vi "Cell TDMS fit and purge MAIN mask v2a BigImage HEATHER 8Bit.vi"() -> ()   [LabVIEW 2020]
uses:
  <vilib>/Utility/file.llb/Read Delimited Spreadsheet (I64).vi
  <vilib>/Utility/file.llb/Write Delimited Spreadsheet (DBL).vi
  <vilib>/Analysis/1siggen.llb/Ramp Pattern by Delta.vi
  <vilib>/Analysis/NI_AALBase.lvlib
  <vilib>/Analysis/NI_AALPro.lvlib
panel:
  in  "Save as binary?":bool
  in  "Min size":u16=400
  out "low threshold":dbl
  in  "threshold 2":dbl(knob)=0.2050666550953167 scale=0.0..1.0
  in  "Save mask?":bool
  in  "WRITE: tiff mask":path=path "F:/Andrey/Heather puncta/Heather mask.tif"
  in  "WRITE: file path to save low/high threshold":path=path "F:/Andrey/Heather puncta/Heather low high threshold.lvm"
  in  "WRITE: file path to save corrected results":path=path "F:/Andrey/Heather puncta/Heather corrected results.lvm"
  in  "Exclude puncta?":bool
  in  "Save centroid results?":bool
  in  "WRITE: file path to save centroid results":path=path "F:/Andrey/Heather puncta/Heather centroid result.lvm"
  out "Fit result picture":picture
  in  "Save PNG?":bool
  in  "WRITE: Fit result save path":path=path "F:/Andrey/Heather puncta/Heather line fit to ave.png"
  out "Fit to data":cluster{"Ramp Pattern":dbl[], dbl[]}[](graph)
  in  "Save corrected?":bool
  in  "WRITE: corrected data file":path=path "F:/Andrey/Heather puncta/Heather cell corrected.tif"
  out "size(s)":i32[](array[numeric])
  in  "Save results?":bool
  in  "WRITE: file path to save results":path=path "F:/Andrey/Heather puncta/Heather results.lvm"
  in  "Use mask?":bool
  in  "READ: Folder/file path for individual cell(s) signal":path=path "E:/WORK/Ehrhardt Lab/Heather Meyer/Txt files for Andrey/phm5S-SUF4 5S variant 4/phm5S_4_cell1"
  out "filename":string
  out "sum":u32
  out "Histogram Graph":T1(graph)
  out "Mask":u8[][](graph)
  out "high threshold":u16
  out "Binarized":u8[][](graph)
  out "new picture (in 8 bit for visualization only)":picture
  in  "Data format?":i8(knob)=1 scale=0.0..2.0
  in  "threshold":dbl(knob)=0.2050666550953167 scale=0.0..1.0
  # "Use mask ON = keep only centroid\nExclude puncta ON = puncta EXCLUDED for the purpose of \ncalculating the curve for image normalization\nCorrected image is cropped by mask INCLUDING puncta,\nregardless of this selector"
  # "txt"
  # "Select file (1 cell only) or folder (for batch processing):"
  # "Version 2.5\nAVM"
  # "120 should be good"
  # "binary"
  # "tiff"
  # "Raw data"
  # "(x100% of max value)"
  # "200-600"
  # "Single Z-section to\nshow for visualization."
  # "Values of intensity for every pixel"
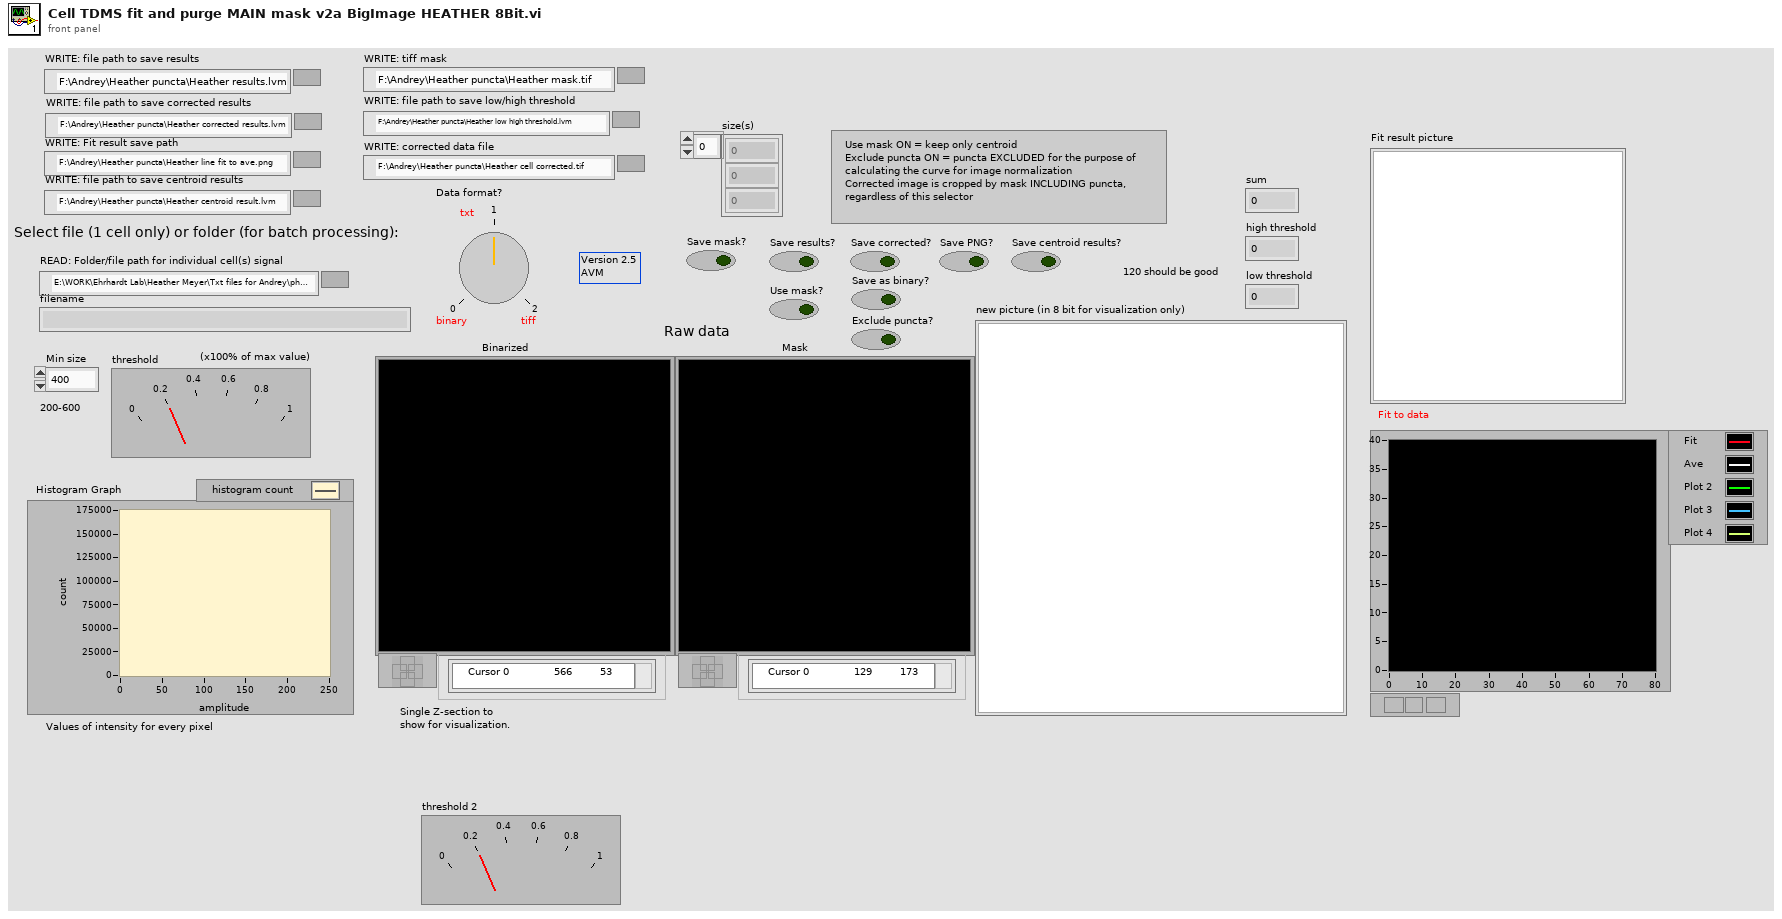
[diagram p1: front panel]
types:
  T1 = cluster{"X Values":dbl[], "Histogram: h(x)":i32[]}
  T2 = cluster{"Width":u16, "Style":enum32{"Solid", "Dash", "Dot", "DashDot", "DashDotDot"}}
  T3 = typedef "imagedata.ctl" = cluster{"image type":i32, "image depth":i32, "image":u8[], "mask":u8[], "colors":u32[], "Rectangle":cluster{"left":i16, "top":i16, "right":i16, "bottom":i16}}
  T4 = typedef "Image Type" = u32
  T5 = typedef "IMAQ Image.ctl" = refnum<image>
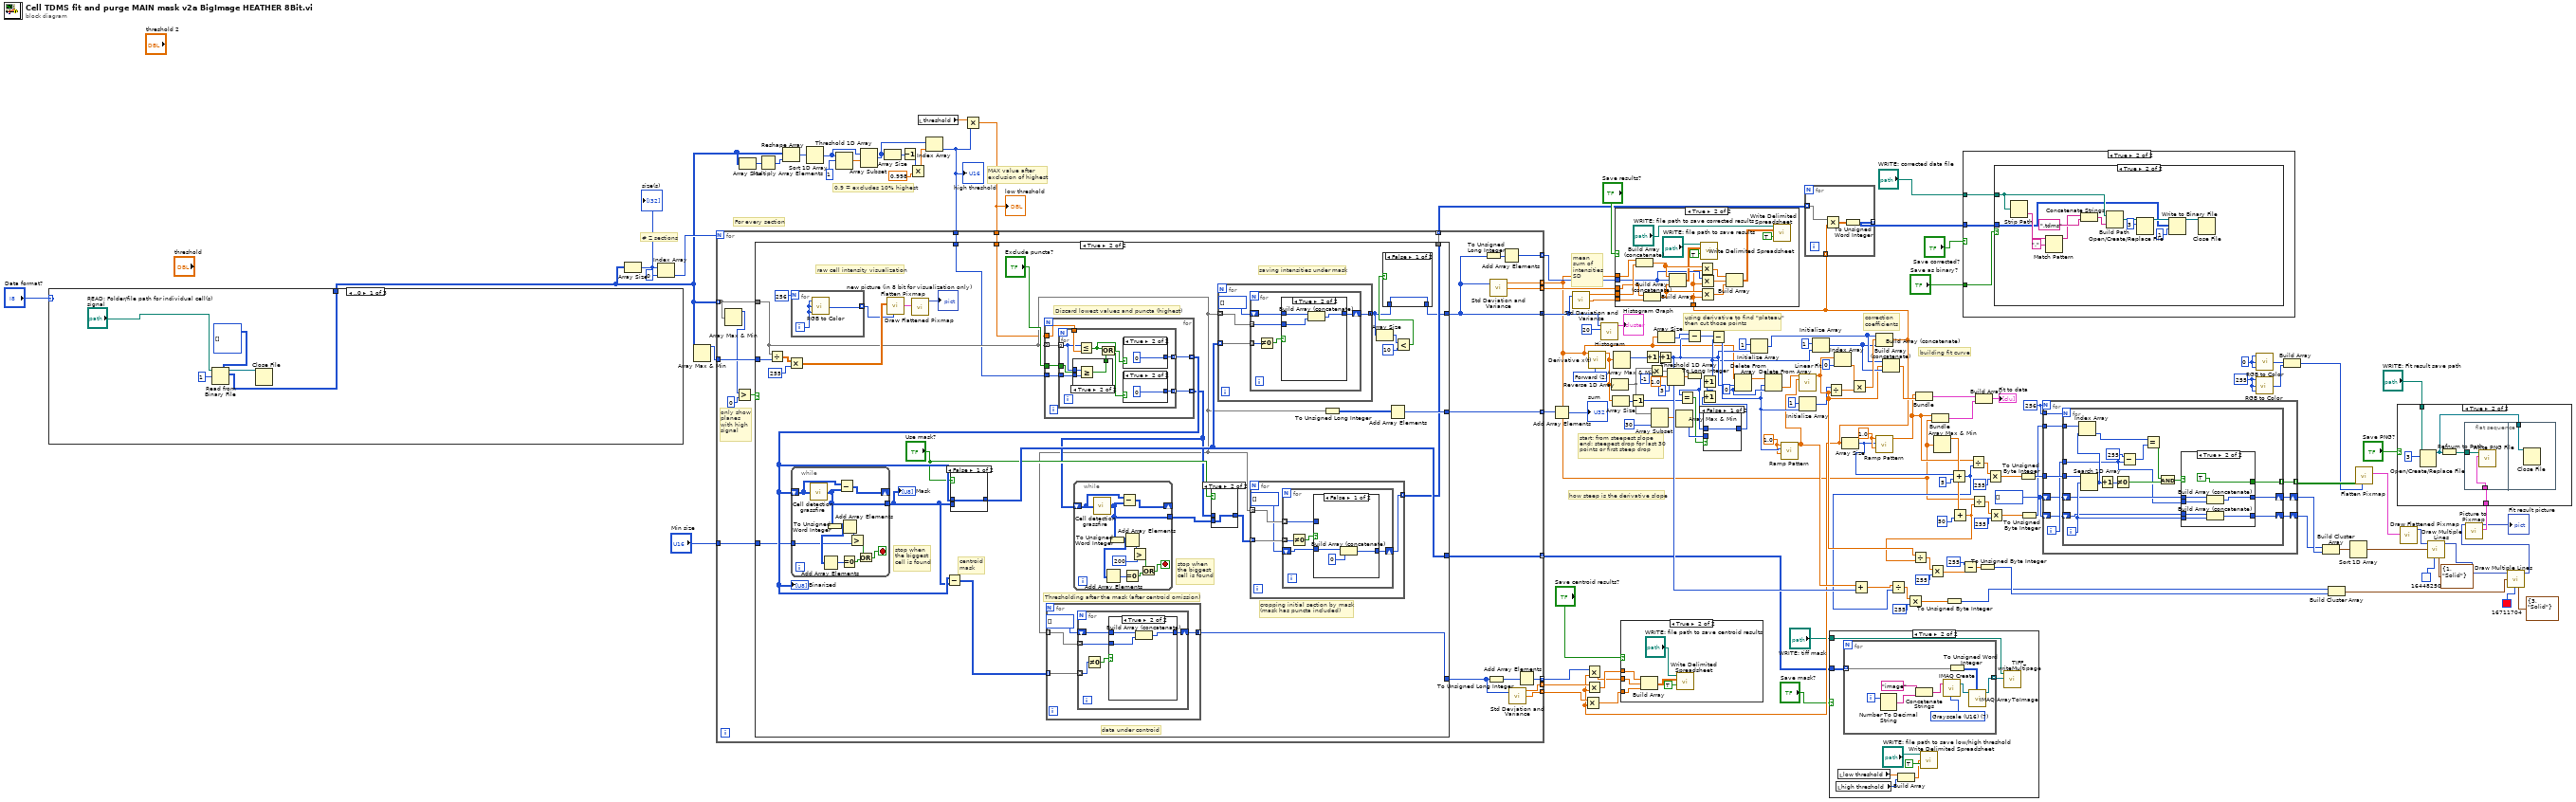
[diagram p0: block diagram]
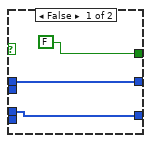
[diagram p5: hidden frame]
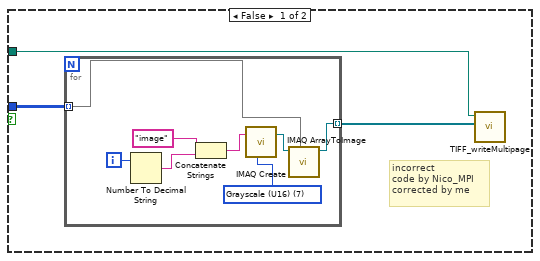
[diagram p8: hidden frame]
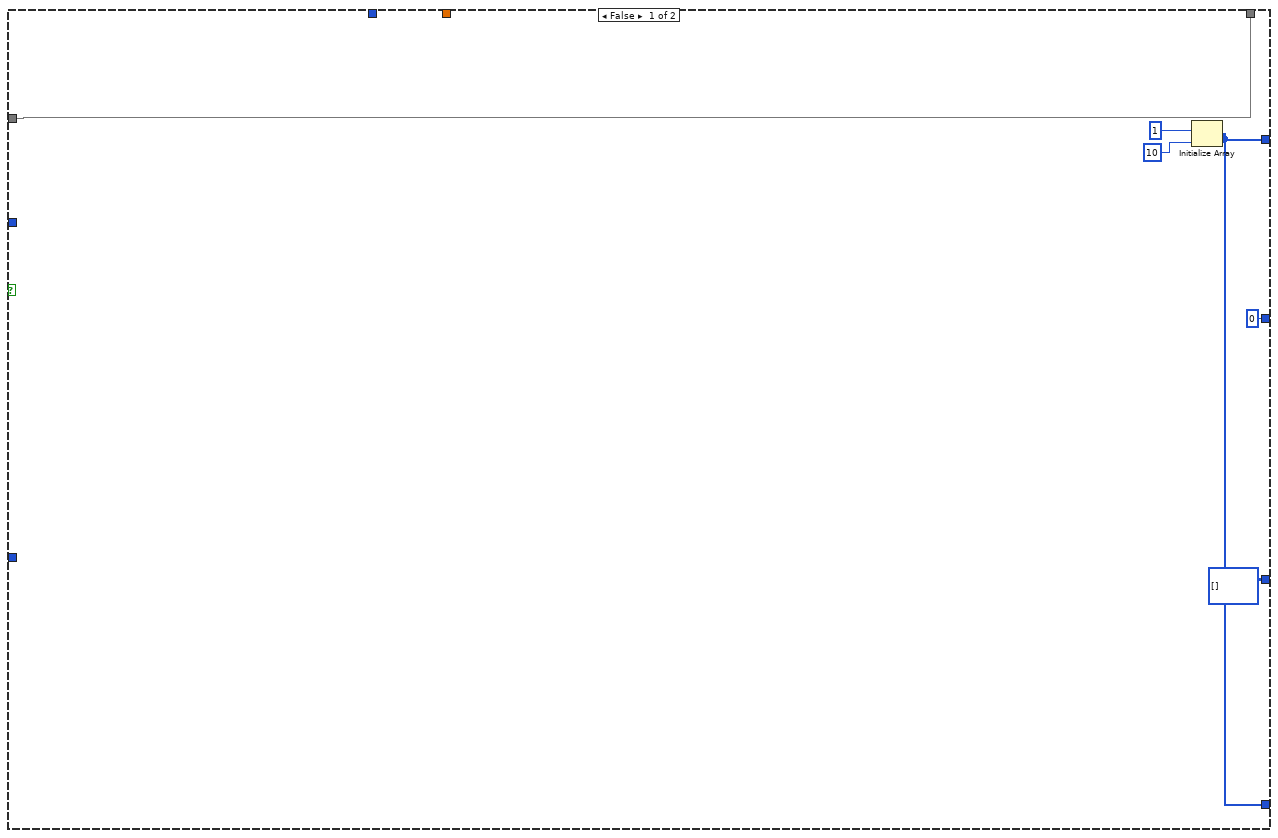
[diagram p10: hidden frame]
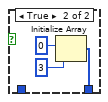
[diagram p11: hidden frame]
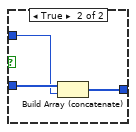
[diagram p12: hidden frame]
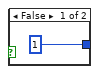
[diagram p17: hidden frame]
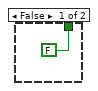
[diagram p18: hidden frame]
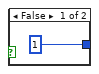
[diagram p19: hidden frame]
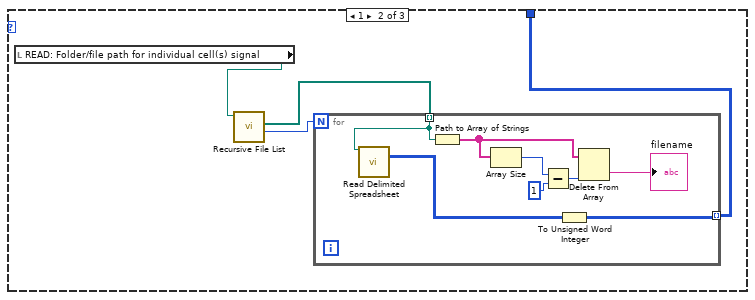
[diagram p20: hidden frame]
diagram:
  w88 = i32[] []
  w66 = u8 255 ("index (row)")
  w78 = u8 0 ("index (row)")
  w95 = 256
  w114 = 1.0 ("delta")
  w117 = 1.0 ("delta")
  w121 = 0 ("index")
  w132 = u16 2 items=["2nd Order Central", "4th Order Central", "Forward", "Backward"] ("method")
  # "building fit curve"
  # "how steep is the derivative slope"
  # "MAX value after\nexclusion of highest"
  # "0.9 = excludes 10% highest"
  # "start: from steepest slope\nend: steepest drop for last 30\npoints or first steep drop"
  # "correction\ncoefficients"
  # "using derivative to find \"plateau\"\nthen cut those points"
  # "For every section"
  # "mean\nsum of\nintensities\nSD"
  # "# Z sections"
  n1 = case shown="..0" "Data format?" {
    tunnel: [w146 w151 w163] -> w9
    frame ..0 {
      n2 = Read from Binary File(5:u8[][][] [] ("subarray"), 9:1, 11:"READ: Folder/file path for individual cell(s) signal") -> (2:w146:u8[][][], 3:w149:refnum<file>)  [unwired: 3 in, 2 out]
      n3 = Close File(refnum=w149) -> ()  [unwired: 1 in, 2 out]
    }
    frame 1 {
      n4 = local read "READ: Folder/file path for individual cell(s) signal"() -> (w150:path)
      n5 = call <vilib>:"Recursive File List.vi"("Folder Path"=w150) -> ("Number of Files"=w153:i32, "All Files in Dir"=w152:path[])  [unwired: 6 in, 3 out]
      n6 = for {
        N: w153 -> [_]
        tunnel: w152 -> [w160] mode=indexing
        tunnel: [w155] -> w151 mode=indexing
        n7 = call-poly <vilib>:"Read Delimited Spreadsheet.vi"("file path (dialog if empty)"=w160) -> ("all rows"=w154:i64[][])  [unwired: 9 in, 5 out]
        n8 = Path to Array of Strings(0:w160) -> (2:w161:string[])  [unwired: 1 out]
        n9 = Array Size(array=w161) -> (size(s)=w156:i32)
        n10 = Subtract(x=w156, y=1 ("index (row)")) -> (x-y=w157:i32)
        n11 = To Unsigned Word Integer(number=w154) -> (unsigned 16bit integer=w155:u16[][])
        n12 = Delete From Array(array=w161, index=w157) -> (deleted portion=→"filename":string)  [unwired: 1 in, 1 out]
      }
    }
    frame 2.. {
      n13 = local read "READ: Folder/file path for individual cell(s) signal"() -> (w164:path)
      n14 = call "Load 3D tiff stack.vi"("Image File"=w164) -> ("24-bit pixmap"=w162:u32[][][])
      n15 = To Unsigned Word Integer(number=w162) -> (unsigned 16bit integer=w163:u16[][][])
    }
  }
  n16 = Array Size(array=w9) -> (size(s)=w143:i32[])
  "size(s)" <- w143
  n17 = Index Array(array=w143, index=0) -> (element=w138:i32)
  n18 = Array Max & Min(array=w9) -> (max value=w139:u16)  [unwired: 3 out]
  n19 = Array Size(array=w9) -> (size(s)=w12:i32[])
  n20 = Multiply Array Elements(1:w12) -> (0:w11:i32)
  n21 = Reshape Array(w9, w11) -> (w16:u16[])
  n22 = Sort 1D Array(array=w16) -> (sorted array=w15:u16[])
  n23 = Threshold 1D Array(2:i16 1 ("y"), 3:w15) -> (0:w17:dbl)  [unwired: 1 in]
  n24 = Array Subset(array=w15, index=w17) -> (w14:u16[])  [unwired: 1 in]
  n25 = Array Size(array=w14) -> (size(s)=w19:i32)
  n26 = Decrement(x=w19) -> (x-1=w18:i32)
  n27 = Multiply(x=w18, y=0.998) -> (x*y=w20:dbl)
  n28 = local read "threshold"() -> (w10:dbl)
  n29 = Index Array(array=w14, index=w20) -> (element=w7:u16)
  "high threshold" <- w7
  n30 = Multiply(x=w10, y=w7) -> (x*y=w8:dbl)
  "low threshold" <- w8
  n31 = for {
    N: w138 -> [_]
    tunnel: [w166] -> w39 mode=concatenating
    tunnel: w139 -> [w185]
    tunnel: w9 -> [w184] mode=indexing
    tunnel: [w180] -> w6 mode=indexing
    tunnel: [w179] -> w136 mode=indexing
    tunnel: [w177] -> w135 mode=indexing
    tunnel: [w176] -> w134 mode=indexing
    tunnel: [w174] -> w38 mode=indexing
    tunnel: [w172] -> w48 mode=indexing
    tunnel: [w171] -> w49 mode=indexing
    tunnel: [w170] -> w35 mode=indexing
    tunnel: [w169] -> w33 mode=indexing
    tunnel: w8 -> [w168]
    tunnel: w7 -> [w167]
    tunnel: "Min size" -> [w165]
    # "only show\nplanes\nwith high\nsignal"
    n32 = Array Max & Min(array=w184) -> (max value=w181:u16)  [unwired: 3 out]
    n33 = Greater?(x=w181, y=i16 0) -> (0:w183:bool)
    n34 = case shown="True" w183 {
      tunnel: [w189 w193] -> w166
      tunnel: w185 -> [_ w214]
      tunnel: w184 -> [w187 w201]
      tunnel: [u16 0 ("index (row)") w213] -> w176
      tunnel: [w189 w210] -> w173
      tunnel: [w187 w203] -> w170
      tunnel: [u8[][] [] ("Cell") w207] -> w169
      tunnel: w168 -> [_ w200]
      tunnel: w167 -> [_ w199]
      tunnel: w165 -> [_ w192]
      frame False {
        n35 = Initialize Array(u16 1 ("index (row)"), u8 10 ("index (row)")) -> (w189:u16[])
      }
      frame True {
        # "cropping initial section by mask\n(mask has puncta included)"
        # "stop when\nthe biggest\ncell is found"
        # "data under controid"
        # "centroid\nmask"
        # "Thresholding after the mask (after centroid omission)"
        # "Discard lowest values and puncta (highest)"
        # "stop when\nthe biggest\ncell is found"
        # "raw cell intensity visualization"
        # "saving intensities under mask"
        n36 = Divide(x=w201, y=w214) -> (x/y=w221:dbl[][])
        n37 = Multiply(x=w221, y=i16 255) -> (x*y=w220:dbl[][])
        n38 = for {
          N: 256 ("samples") -> [_]
          tunnel: [w314] -> w217 mode=indexing
          i -> [w315]
          n39 = call <vilib>:"RGB to Color.vi"("B"=w315, "G"=w315, "R"=w315) -> ("Color"=w314:u32)
        }
        n40 = call <vilib>:"Flatten Pixmap.vi"("colors"=w217, "8-bit pixmap"=w220) -> ("image data"=w216:T3)  [unwired: 9 in]
        n41 = call <vilib>:"Draw Flattened Pixmap.vi"("image data"=w216) -> ("new picture"=→"new picture (in 8 bit for visualization only)":picture)  [unwired: 8 in]
        n42 = for {
          tunnel: [w296] -> w212 mode=indexing
          tunnel: w201 -> [w295] mode=indexing
          tunnel: w200 -> [w294]
          tunnel: w199 -> [w293]
          tunnel: "Exclude puncta?" -> [w292]
          tunnel: [w291] -> w205 mode=indexing
          n43 = for {
            tunnel: w295 -> [w300] mode=indexing
            tunnel: [w305] -> w296 mode=indexing
            tunnel: w294 -> [w304]
            tunnel: w293 -> [w301]
            tunnel: w292 -> [w299]
            tunnel: [w297] -> w291 mode=indexing
            n44 = case shown="True" w299 {
              tunnel: [FALSE w311] -> w303
              tunnel: w301 -> [_ w310]
              tunnel: w300 -> [_ w309]
              frame False {
              }
              frame True {
                n45 = Greater Or Equal?(x=w309, y=w310) -> (x >= y?=w311:bool)
              }
            }
            n46 = Less Or Equal?(x=w300, y=w304) -> (x <= y?=w298:bool)
            n47 = Or(x=w298, y=w303) -> (x .or. y?=w302:bool)
            n48 = case shown="True" w302 {
              tunnel: [u8 1 ("index (row)") u8 0 ("index (row)")] -> w305
              frame False {
              }
              frame True {
              }
            }
            n49 = case shown="True" w298 {
              tunnel: [u8 1 ("index (row)") u8 0 ("index (row)")] -> w297
              frame False {
              }
              frame True {
              }
            }
          }
        }
        "Binarized" <- w212
        n50 = while {
          shift-right: [w276] -> _
          shift-left: w212 -> [w277]
          tunnel: [w274] -> w209
          tunnel: w192 -> [w268]
          stop <- w272 stop-if-true
          n51 = call "Cell detection grassfire.vi"("Intensities"=w277) -> ("Cell"=w274:u8[][])
          n52 = To Unsigned Word Integer(number=w274) -> (unsigned 16bit integer=w269:u16[][])
          n53 = Add Array Elements(numeric array=w269) -> (sum=w270:u16)
          n54 = Subtract(x=w277, y=w274) -> (x-y=w276:u8[][])
          n55 = Equal To 0?(x=w270) -> (x = 0?=w271:bool)
          n56 = Add Array Elements(numeric array=w269) -> (sum=w275:u16)
          n57 = Greater?(x=w275, y=w268) -> (0:w273:bool)
          n58 = Or(x=w273, y=w271) -> (x .or. y?=w272:bool)
        }
        "Mask" <- w209
        n59 = Subtract(x=w212, y=w209) -> (x-y=w211:u8[][])
        n60 = case shown="False" "Use mask?" {
          tunnel: w212 -> [w266 _]
          tunnel: [w266 w267] -> w207
          tunnel: w209 -> [_ w267]
          frame False {
          }
          frame True {
          }
        }
        n61 = for {
          tunnel: w201 -> [w255] mode=indexing
          tunnel: w211 -> [w256] mode=indexing
          tunnel: [w253] -> w210 mode=concatenating
          n62 = for {
            tunnel: w256 -> [w260] mode=indexing
            shift-right: [w259] -> w253
            shift-left: u16[] [] -> [w257]
            tunnel: w255 -> [w258] mode=indexing
            n63 = Not Equal To 0?(x=w260) -> (x != 0?=w261:bool)
            n64 = case shown="True" w261 {
              tunnel: w257 -> [w262 w264]
              tunnel: [w262 w263] -> w259
              tunnel: w258 -> [_ w265]
              frame False {
              }
              frame True {
                n65 = Build Array (concatenate)(w264, w265) -> (w263:u16[])
              }
            }
          }
        }
        n66 = while {
          shift-right: [w251] -> _
          shift-left: w205 -> [w252]
          tunnel: [w248] -> w204
          stop <- w246 stop-if-true
          n67 = call "Cell detection grassfire.vi"("Intensities"=w252) -> ("Cell"=w248:u8[][])
          n68 = To Unsigned Word Integer(number=w248) -> (unsigned 16bit integer=w243:u16[][])
          n69 = Add Array Elements(numeric array=w243) -> (sum=w244:u16)
          n70 = Subtract(x=w252, y=w248) -> (x-y=w251:u8[][])
          n71 = Equal To 0?(x=w244) -> (x = 0?=w245:bool)
          n72 = Add Array Elements(numeric array=w243) -> (sum=w250:u16)
          n73 = Greater?(x=w250, y=u16 200) -> (0:w247:bool)
          n74 = Or(x=w247, y=w245) -> (x .or. y?=w246:bool)
        }
        n75 = case shown="True" "Use mask?" {
          tunnel: w205 -> [w241 _]
          tunnel: [w241 w242] -> w202
          tunnel: w204 -> [_ w242]
          frame False {
          }
          frame True {
          }
        }
        n76 = for {
          tunnel: w201 -> [w280] mode=indexing
          tunnel: w207 -> [w281] mode=indexing
          tunnel: [w279] -> w194 mode=concatenating
          n77 = for {
            tunnel: w281 -> [w285] mode=indexing
            shift-right: [w284] -> w279
            shift-left: u16[] [] -> [w282]
            tunnel: w280 -> [w283] mode=indexing
            n78 = Not Equal To 0?(x=w285) -> (x != 0?=w286:bool)
            n79 = case shown="True" w286 {
              tunnel: w282 -> [w287 w290]
              tunnel: [w287 w289] -> w284
              tunnel: w283 -> [_ w288]
              frame False {
              }
              frame True {
                n80 = Build Array (concatenate)(w290, w288) -> (w289:u16[])
              }
            }
          }
        }
        n81 = for {
          tunnel: w201 -> [w228] mode=indexing
          tunnel: w202 -> [w229] mode=indexing
          tunnel: [w226] -> w203 mode=indexing
          n82 = for {
            tunnel: w229 -> [w233] mode=indexing
            tunnel: w228 -> [w232] mode=indexing
            shift-right: [w231] -> w226
            shift-left: u16[] [] -> [w230]
            n83 = Not Equal To 0?(x=w233) -> (x != 0?=w234:bool)
            n84 = case shown="False" w234 {
              tunnel: w232 -> [_ w238]
              tunnel: [w235 w240] -> w231
              tunnel: w230 -> [w236 w239]
              frame False {
                n85 = Build Array (concatenate)(w236, u16 0 ("Numeric")) -> (w235:u16[])
              }
              frame True {
                n86 = Build Array (concatenate)(w239, w238) -> (w240:u16[])
              }
            }
          }
        }
        n87 = To Unsigned Long Integer(number=w201) -> (unsigned 32bit integer=w215:u32[][])
        n88 = Array Size(array=w194) -> (size(s)=w197:i32)
        n89 = Add Array Elements(numeric array=w215) -> (sum=w213:u32)
        n90 = Less?(x=w197, y=u16 10 ("index (row)")) -> (x < y?=w195:bool)
        n91 = case shown="False" w195 {
          tunnel: w194 -> [w222 _]
          tunnel: [w222 w223] -> w193
          frame False {
          }
          frame True {
            n92 = Initialize Array(u16 0 ("index (row)"), u8 3 ("index (row)")) -> (w223:u16[])
          }
        }
      }
    }
    n93 = To Unsigned Long Integer(number=w166) -> (unsigned 32bit integer=w178:u32[])
    n94 = To Unsigned Long Integer(number=w173) -> (unsigned 32bit integer=w175:u32[])
    n95 = call <vilib>:"Std Deviation and Variance.vi"("X"=w166) -> ("mean"=w180:dbl, "standard deviation"=w177:dbl)  [unwired: 1 in, 1 out]
    n96 = Add Array Elements(numeric array=w178) -> (sum=w179:u32)
    n97 = call <vilib>:"Std Deviation and Variance.vi"("X"=w173) -> ("mean"=w172:dbl, "standard deviation"=w171:dbl)  [unwired: 1 in, 1 out]
    n98 = Add Array Elements(numeric array=w175) -> (sum=w174:u32)
  }
  n99 = Add Array Elements(numeric array=w134) -> (sum=→"sum":u32)
  n100 = call <vilib>:"Std Deviation and Variance.vi"("X"=w39) -> ("mean"=w41:dbl, "standard deviation"=w40:dbl)  [unwired: 1 in, 1 out]
  n101 = call <vilib>:"Derivative x(t).vi"("method"=w132, "X"=w6) -> ("dX/dt"=w27:dbl[])  [unwired: 8 in, 1 out]
  n102 = call <vilib>:"Histogram.vi"("intervals"=u8 20 ("index (row)"), "X"=w39) -> ("Histogram Graph"=→"Histogram Graph":T1)  [unwired: 6 in, 3 out]
  n103 = Reverse 1D Array(array=w27) -> (reversed array=w30:dbl[])
  n104 = Array Size(array=w27) -> (size(s)=w28:i32)
  n105 = Array Max & Min(array=w27) -> (max index (indices)=w61:i32)  [unwired: 3 out]
  n106 = Decrement(x=w28) -> (x-1=w3:i32)
  n107 = Increment(x=w61) -> (x+1=w60:i32)
  n108 = Multiply(x=w30, y=i8 -1 ("index (row)")) -> (x*y=w31:dbl[])
  n109 = Array Subset(array=w30, length=30 ("index")) -> (w44:dbl[])  [unwired: 1 in]
  n110 = Increment(x=w60) -> (x+1=w58:i32)
  n111 = Array Size(array=w6) -> (size(s)=w131:i32)
  n112 = Threshold 1D Array(1:3 ("start index (0)"), 2:1.0 ("y"), 3:w31) -> (0:w25:dbl)
  n113 = Array Max & Min(array=w44) -> (min index (indices)=w43:i32)  [unwired: 3 out]
  n114 = Subtract(x=w131, y=w58) -> (x-y=w130:i32)
  n115 = To Long Integer(number=w25) -> (32bit integer=w2:i32)
  n116 = Equal?(x=w2, y=w3) -> (x = y?=w26:bool)
  n117 = case shown="False" w26 {
    tunnel: w2 -> [w316 _]
    tunnel: w43 -> [_ w317]
    tunnel: [w316 w317] -> w42
    frame False {
    }
    frame True {
    }
  }
  n118 = Increment(x=w42) -> (x+1=w24:i32)
  n119 = Increment(x=w24) -> (x+1=w23:i32)
  n120 = Subtract(x=w130, y=w23) -> (x-y=w118:i32)
  n121 = Delete From Array(array=w6, length=w58, index=w121) -> (array with subset deleted=w120:dbl[])  [unwired: 1 out]
  n122 = Initialize Array(u8 1 ("index (row)"), w58) -> (w113:u8[])
  n123 = Delete From Array(array=w120, length=w118, index=w121) -> (deleted portion=w119:dbl[])  [unwired: 1 out]
  n124 = call-poly <vilib>:"Ramp Pattern.vi"("start"=w117, "end"=w118, "delta"=w117) -> ("Ramp Pattern"=w62:dbl[])  [unwired: 6 in, 2 out]
  n125 = call <vilib>:"Linear Fit.vi"("Y"=w119, "X"=w62) -> ("Best Linear Fit"=w69:dbl[])  [unwired: 9 in, 4 out]
  n126 = Initialize Array(u8 1 ("index (row)"), w118) -> (w126:u8[])
  n127 = Initialize Array(u8 1 ("index (row)"), w23) -> (w112:u8[])
  n128 = Divide(x=w126, y=w69) -> (x/y=w111:dbl[])
  n129 = case shown="True" "Save mask?" {
    tunnel: "WRITE: tiff mask" -> [_ w324]
    tunnel: w33 -> [_ w323]
    frame False {
    }
    frame True {
      n130 = local read "high threshold"() -> (w320:u16)
      n131 = local read "low threshold"() -> (w319:dbl)
      n132 = for {
        tunnel: w323 -> [w327] mode=indexing
        tunnel: [w328] -> w325 mode=indexing
        i -> [w329]
        w333 = T4 7 items=["Grayscale (U8)", "Grayscale (I16)", "Grayscale (SGL)", "Complex (CSG)", "RGB (U32)", "HSL (U32)", "RGB (U64)", "Grayscale (U16)"] ("Image Type")
        n133 = Number To Decimal String(number=w329) -> (decimal integer string=w331:string)  [unwired: 1 in]
        n134 = Concatenate Strings("image" ("name or relative path"), w331) -> (w330:string)
        n135 = call "IMAQ Create"("Image Name"=w330, "Image Type"=w333) -> ("New Image"=w334:T5)  [unwired: 3 in, 1 out]
        n136 = To Unsigned Word Integer(number=w327) -> (unsigned 16bit integer=w326:u16[][])
        n137 = call "IMAQ ArrayToImage"("Image Pixels (U16)"=w326, "Image"=w334) -> ("Image Out"=w328:T5)  [unwired: 8 in, 1 out]
      }
      n138 = Build Array(w319, w320) -> (w318:dbl[])
      n139 = call-poly <vilib>:"Write Delimited Spreadsheet.vi"("file path (dialog if empty)"="WRITE: file path to save low/high threshold", "1D data"=w318, "append to file? (new file:F)"=TRUE) -> ()  [unwired: 11 in, 2 out]
      n140 = call "TIFF_writeMultipage.vi"("Array in"=w325, "file (use dialog)"=w324) -> ()  [unwired: 9 in, 1 out]
    }
  }
  n141 = Index Array(array=w69, index=0) -> (element=w124:dbl)
  n142 = Multiply(x=w124, y=w111) -> (x*y=w116:dbl[])
  n143 = Add(x=w62, y=w58) -> (x+y=w63:dbl[])
  n144 = Build Array (concatenate)(w113, w116, w112) -> (w36:dbl[])
  n145 = Multiply(x=w49, y=w36) -> (x*y=w46:dbl[])
  n146 = Multiply(x=w38, y=w36) -> (x*y=w37:dbl[])
  n147 = Multiply(x=w48, y=w36) -> (x*y=w47:dbl[])
  n148 = case shown="True" "Save results?" {
    tunnel: w6 -> [_ w349]
    tunnel: w136 -> [_ w341]
    tunnel: w135 -> [_ w347]
    tunnel: w41 -> [_ w348]
    tunnel: w40 -> [_ w346]
    tunnel: w36 -> [_ w339]
    frame False {
    }
    frame True {
      n149 = Build Array (concatenate)(w349, w348) -> (w343:dbl[])
      n150 = Build Array (concatenate)(w347, w346) -> (w340:dbl[])
      n151 = Build Array(w343, w341, w340) -> (w342:dbl[][])
      n152 = Multiply(x=w343, y=w339) -> (x*y=w338:dbl[])
      n153 = Multiply(x=w341, y=w339) -> (x*y=w337:dbl[])
      n154 = Multiply(x=w340, y=w339) -> (x*y=w336:dbl[])
      n155 = call-poly <vilib>:"Write Delimited Spreadsheet.vi"("file path (dialog if empty)"="WRITE: file path to save results", "2D data"=w342, "append to file? (new file:F)"=TRUE) -> ()  [unwired: 11 in, 2 out]
      n156 = Build Array(w338, w337, w336) -> (w335:dbl[][])
      n157 = call-poly <vilib>:"Write Delimited Spreadsheet.vi"("file path (dialog if empty)"="WRITE: file path to save corrected results", "2D data"=w335, "append to file? (new file:F)"=TRUE) -> ()  [unwired: 11 in, 2 out]
    }
  }
  n158 = case shown="True" "Save centroid results?" {
    tunnel: w37 -> [_ w353]
    tunnel: w47 -> [_ w352]
    tunnel: w46 -> [_ w354]
    frame False {
    }
    frame True {
      n159 = Build Array(w352, w353, w354) -> (w357:dbl[][])
      n160 = call-poly <vilib>:"Write Delimited Spreadsheet.vi"("file path (dialog if empty)"="WRITE: file path to save centroid results", "2D data"=w357, "append to file? (new file:F)"=TRUE) -> ()  [unwired: 11 in, 2 out]
    }
  }
  n161 = for {
    tunnel: w35 -> [w361] mode=indexing
    tunnel: w36 -> [w360] mode=indexing
    tunnel: [w358] -> w115 mode=indexing
    n162 = Multiply(x=w361, y=w360) -> (x*y=w359:dbl[][])
    n163 = To Unsigned Word Integer(number=w359) -> (unsigned 16bit integer=w358:u16[][])
  }
  n164 = Array Size(array=w36) -> (size(s)=w97:i32)
  n165 = call-poly <vilib>:"Ramp Pattern.vi"("start"=w114, "end"=w97, "delta"=w114) -> ("Ramp Pattern"=w96:dbl[])  [unwired: 6 in, 2 out]
  n166 = Build Array (concatenate)(w113, w69, w112) -> (w110:dbl[])
  n167 = Bundle("Ramp Pattern"=w96, w110) -> (w109:cluster{"Ramp Pattern":dbl[], dbl[]})  [unwired: 1 in]
  n168 = Bundle("Ramp Pattern"=w96, w6) -> (w108:cluster{"Ramp Pattern":dbl[], dbl[]})  [unwired: 1 in]
  n169 = Array Max & Min(array=w6) -> (max value=w103:dbl)  [unwired: 3 out]
  n170 = Add(x=w97, y=u16 5 ("index (row)")) -> (x+y=w51:i32)
  n171 = Divide(x=w63, y=w51) -> (x/y=w67:dbl[])
  n172 = Multiply(x=w67, y=u16 255 ("index (row)")) -> (x*y=w54:dbl[])
  n173 = To Unsigned Byte Integer(number=w54) -> (unsigned 8bit integer=w53:u8[])
  n174 = Add(x=w103, y=u16 50 ("index (row)")) -> (x+y=w50:dbl)
  n175 = Divide(x=w69, y=w50) -> (x/y=w70:dbl[])
  n176 = Multiply(x=w70, y=u16 255 ("index (row)")) -> (x*y=w64:dbl[])
  n177 = Subtract(x=u16 255, y=w64) -> (x-y=w56:dbl[])
  n178 = case shown="True" "Save corrected?" {
    tunnel: "WRITE: corrected data file" -> [_ w363]
    tunnel: w115 -> [_ w364]
    tunnel: "Save as binary?" -> [_ w362]
    frame False {
    }
    frame True {
      n179 = case shown="True" w362 {
        tunnel: w364 -> [w366 w376]
        tunnel: w363 -> [w365 w381]
        frame False {
          # "incorrect\ncode by Nico_MPI\ncorrected by me"
          n180 = for {
            tunnel: w366 -> [w368] mode=indexing
            tunnel: [w369] -> w367 mode=indexing
            i -> [w370]
            w374 = T4 7 items=["Grayscale (U8)", "Grayscale (I16)", "Grayscale (SGL)", "Complex (CSG)", "RGB (U32)", "HSL (U32)", "RGB (U64)", "Grayscale (U16)"] ("Image Type")
            n181 = Number To Decimal String(number=w370) -> (decimal integer string=w372:string)  [unwired: 1 in]
            n182 = Concatenate Strings("image" ("name or relative path"), w372) -> (w371:string)
            n183 = call "IMAQ Create"("Image Name"=w371, "Image Type"=w374) -> ("New Image"=w375:T5)  [unwired: 3 in, 1 out]
            n184 = call "IMAQ ArrayToImage"("Image Pixels (U16)"=w368, "Image"=w375) -> ("Image Out"=w369:T5)  [unwired: 8 in, 1 out]
          }
          n185 = call "TIFF_writeMultipage.vi"("Array in"=w367, "file (use dialog)"=w365) -> ()  [unwired: 9 in, 1 out]
        }
        frame True {
          n186 = Strip Path(path=w381) -> (name=w379:string)  [unwired: 1 out]
          n187 = Match Pattern(string=w379, regular expression=".") -> (before substring=w377:string)  [unwired: 1 in, 3 out]
          n188 = Concatenate Strings(w377, ".tdms" ("name or relative path")) -> (w382:string)
          n189 = Build Path(base path=w381, name or relative path=w382) -> (appended path=w385:path)
          n190 = Open/Create/Replace File(file path (use dialog)=w385, operation (0:open)=3) -> (refnum out=w386:refnum<file>)  [unwired: 4 in, 2 out]
          n191 = Write to Binary File(file (use dialog)=w386, data=w376, 9:1) -> (refnum out=w387:refnum<file>)  [unwired: 3 in, 2 out]
          n192 = Close File(refnum=w387) -> ()  [unwired: 1 in, 2 out]
        }
      }
    }
  }
  n193 = Divide(x=w96, y=w51) -> (x/y=w98:dbl[])
  n194 = Divide(x=w6, y=w50) -> (x/y=w101:dbl[])
  n195 = Build Array(w109, w108) -> (→"Fit to data":cluster{"Ramp Pattern":dbl[], dbl[]}[])
  n196 = To Unsigned Byte Integer(number=w56) -> (unsigned 8bit integer=w55:u8[])
  n197 = Multiply(x=w98, y=u16 255 ("index (row)")) -> (x*y=w52:dbl[])
  n198 = Multiply(x=w101, y=u16 255 ("index (row)")) -> (x*y=w57:dbl[])
  n199 = To Unsigned Byte Integer(number=w52) -> (unsigned 8bit integer=w94:u8[])
  n200 = To Unsigned Byte Integer(number=w57) -> (unsigned 8bit integer=w90:u8[])
  n201 = for {
    N: w95 -> [_]
    tunnel: w95 -> [w396]
    tunnel: w94 -> [w395]
    tunnel: [w394] -> w93 mode=indexing
    tunnel: w90 -> [w393]
    shift-right: [w391] -> w82
    shift-left: w88 -> [w390]
    shift-right: [w389] -> w81
    shift-left: w88 -> [w388]
    i -> [w392]
    n202 = for {
      N: w396 -> [_]
      tunnel: w395 -> [w408]
      tunnel: [w413] -> w394 mode=indexing
      tunnel: w393 -> [w412]
      tunnel: w392 -> [w397]
      shift-right: [w403] -> w391
      shift-left: w390 -> [w402]
      shift-right: [w401] -> w389
      shift-left: w388 -> [w400]
      i -> [w404]
      n203 = Search 1D Array(1D array=w408, element=w404) -> (index of element=w405:i32)  [unwired: 1 in]
      n204 = Index Array(array=w412, index=w405) -> (element=w411:u8)
      n205 = Increment(x=w405) -> (x+1=w407:i32)
      n206 = Not Equal To 0?(x=w407) -> (x != 0?=w406:bool)
      n207 = Subtract(x=255, y=w397) -> (x-y=w398:i32)
      n208 = Equal?(x=w411, y=w398) -> (x = y?=w409:bool)
      n209 = And(x=w409, y=w406) -> (x .and. y?=w410:bool)
      n210 = case shown="True" w410 {
        tunnel: [FALSE TRUE] -> w413
        tunnel: w404 -> [_ w420]
        tunnel: w397 -> [_ w422]
        tunnel: [w415 w419] -> w403
        tunnel: w402 -> [w415 w421]
        tunnel: [w414 w418] -> w401
        tunnel: w400 -> [w414 w417]
        frame False {
        }
        frame True {
          n211 = Build Array (concatenate)(w421, w422) -> (w419:i32[])
          n212 = Build Array (concatenate)(w417, w420) -> (w418:i32[])
        }
      }
    }
  }
  n213 = call <vilib>:"RGB to Color.vi"("B"=w66, "G"=w66, "R"=w66) -> ("Color"=w91:u32)
  n214 = call <vilib>:"RGB to Color.vi"("B"=w78, "G"=w78, "R"=w78) -> ("Color"=w92:u32)
  n215 = Build Array(w92, w91) -> (w87:u32[])
  n216 = Build Cluster Array(w81, w82) -> (w80:cluster{i32, i32}[])
  n217 = Build Cluster Array(w53, w55) -> (w74:cluster{u8, u8}[])
  n218 = Sort 1D Array(array=w80) -> (sorted array=w79:cluster{i32, i32}[])
  n219 = call <vilib>:"Flatten Pixmap.vi"("colors"=w87, "1-bit pixmap"=w93) -> ("image data"=w89:T3)  [unwired: 9 in]
  n220 = call <vilib>:"Draw Flattened Pixmap.vi"("image data"=w89) -> ("new picture"=w86:picture)  [unwired: 8 in]
  n221 = call <vilib>:"Draw Multiple Lines.vi"("picture"=w86, "line endpoints"=w79, "color(black)"=u32 16448250, "pen"=T2 {"Width"=1, "Style"=enum."Solid"}) -> ("new picture"=w73:picture)  [unwired: 5 in]
  n222 = call <vilib>:"Draw Multiple Lines.vi"("picture"=w73, "line endpoints"=w74, "color(black)"=u32 16711704, "pen"=T2 {"Width"=3, "Style"=enum."Solid"}) -> ("new picture"=w72:picture)  [unwired: 5 in]
  n223 = call <vilib>:"Picture to Pixmap.vi"("picture"=w72) -> ("image data"=w85:T3, "new picture"=→"Fit result picture":picture)  [unwired: 9 in]
  n224 = case shown="True" "Save PNG?" {
    tunnel: "WRITE: Fit result save path" -> [_ w428]
    tunnel: w85 -> [_ w424]
    frame False {
    }
    frame True {
      n225 = Open/Create/Replace File(file path (use dialog)=w428, operation (0:open)=u16 3 ("index (row)")) -> (refnum out=w425:refnum<file>)  [unwired: 4 in, 2 out]
      n226 = Refnum to Path(1:w425) -> (0:w426:path)
      n227 = flat-sequence {
        tunnel: w426 -> [w430]
        tunnel: w424 -> [w429]
        tunnel: w425 -> [w431]
        frame #0 {
          n228 = call <vilib>:"Write PNG File.vi"("image data"=w429, "path to PNG file"=w430) -> ()  [unwired: 8 in, 2 out]
        }
        frame #1 {
          n229 = Close File(refnum=w431) -> ()  [unwired: 1 in, 2 out]
        }
      }
    }
  }
